vi "Configure Trigger (Current).vi"(6 "Settle (1mS)":u32=1, 8 "error in (no error)":errorcluster, 10 "Triggering Value (0)":dbl, 11 "VISA resource name":refnum<visa-resource-name>) -> (0 "error out":errorcluster, 3 "VISA resource name out":refnum<visa-resource-name>)   [LabVIEW 2012, in "TDK-Lambda Z.lvlib"]
doc: "Configures (Fix mode) output control, each triggered output voltage or current value is explicitly specified by a triggered-level command (for example, CURR:TRIG 1.55). The trigger then causes the output to change to this pending triggered level."
uses:
  TDK-Lambda Z.lvlib
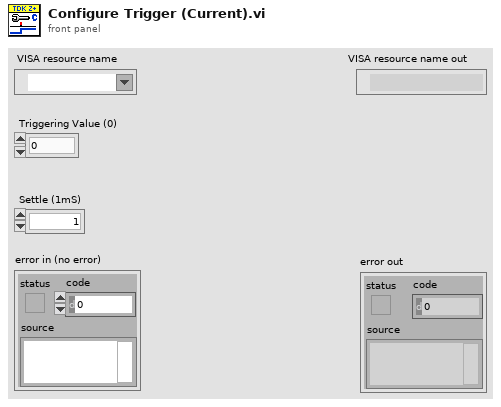
[diagram p1: front panel]
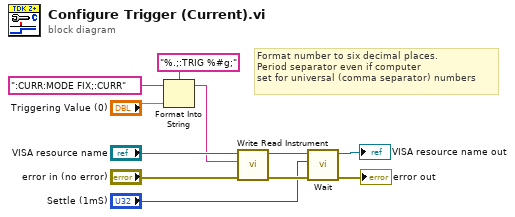
[diagram p0: block diagram]
diagram:
  # "Format number to six decimal places.\nPeriod separator even if computer \nset for universal (comma separator) numbers"
  n1 = Format Into String(format string="%.;:TRIG %#g;", initial string=":CURR:MODE FIX;:CURR" ("concatenated string"), "Triggering Value (0)") -> (resulting string=w4:string)  [unwired: 1 in, 1 out]
  n2 = call "Write Read Instrument.vi"("error in (no error)"="error in (no error)", "SCPI  Write Command/Query"=w4, "VISA resource name"="VISA resource name") -> ("error out"=w8:errorcluster, "VISA resource name out"=w9:refnum<visa-resource-name>)  [unwired: 6 in, 1 out]
  n3 = call "Wait.vi"("error in (no error)"=w8, "Wait (1mS)"="Settle (1mS)", "VISA resource name"=w9) -> ("error out"=→"error out":errorcluster, "VISA resource name out"=→"VISA resource name out":refnum<visa-resource-name>)  [unwired: 7 in]
